vi "Get SubVI RefNum.vi"(8 "error in (no error)":errorcluster, 11 "xceSubPanel in":refnum<class "xceSubPanel.lvclass">) -> (0 "error out":errorcluster, 2 "subVI*":refnum<vi>, 3 "xceSubPanel out":refnum<class "xceSubPanel.lvclass">)   [LabVIEW 2013, in "xceSubPanel.lvclass"]
uses:
  xceSubPanel.lvclass
  xceSubPanel.lvclass/xceSubPanel.ctl
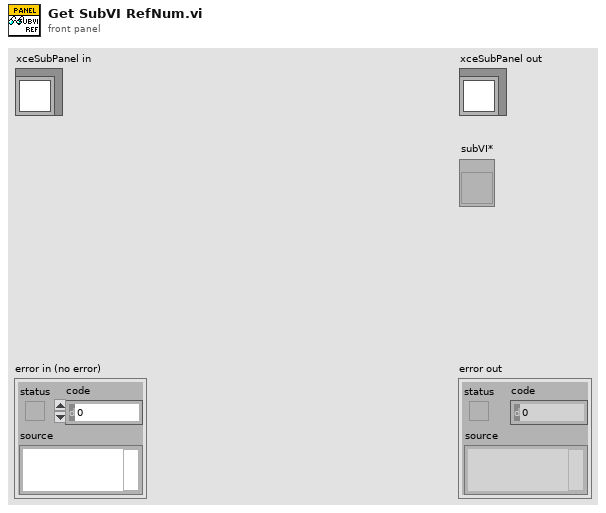
[diagram p1: front panel]
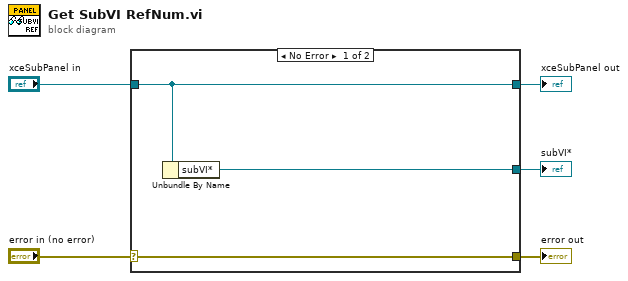
[diagram p0: block diagram]
diagram:
  n1 = case shown="No Error" "error in (no error)" {
    selector: "error in (no error)" -> [w8 w9]
    tunnel: [w8 w9] -> w4
    tunnel: [w7 w10] -> w2
    tunnel: "xceSubPanel in" -> [w7 w10]
    tunnel: [w6 _] -> w1
    frame No Error {
      n2 = Unbundle By Name(w7) -> ("subVI*"=w6:refnum<vi>)
    }
    frame Error {
    }
  }
  "error out" <- w4
  "xceSubPanel out" <- w2
  "subVI*" <- w1
